vi "SwerveJoystickRotationScaling.vi"(2 "Rotation Scaling":dbl(slide)=2.0 min=1.0 max=4.0 scale=1.0..4.0, 3 "Rotation Deadband":dbl(slide)=0.05 min=0.0 max=0.4 scale=0.0..0.4, 4 "Auto Control":bool, 5 "Raw Rotation Joystick":dbl) -> (0 "Scaled Rotation Joystick":dbl, 1 "In Deadband":bool)   [LabVIEW 2019]
doc: "Applies a deadband and nonlinear scaling to the rotation axis of a swerve drive. Includes a hook to override the non-linear deadband and scaling when the rotation is under autonomous control."
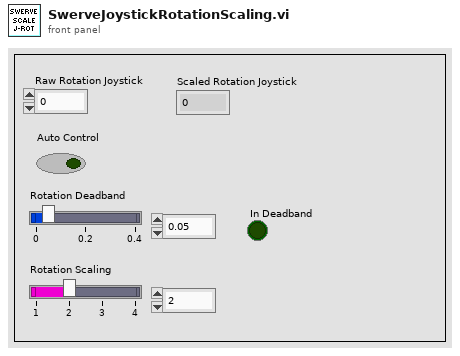
[diagram p1: front panel]
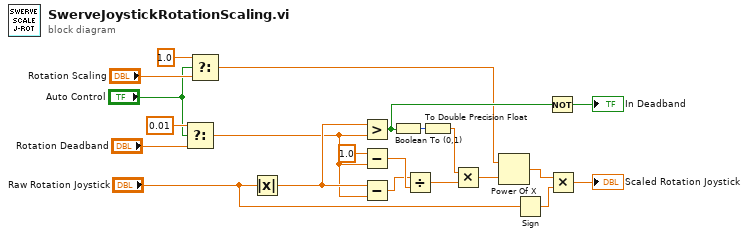
[diagram p0: block diagram]
diagram:
  n1 = Select(t=0.01, s="Auto Control", f="Rotation Deadband") -> (s? t:f=w5:dbl)
  n2 = Select(t=1.0, s="Auto Control", f="Rotation Scaling") -> (s? t:f=w2:dbl)
  n3 = Absolute Value(x="Raw Rotation Joystick") -> (abs(x)=w17:dbl)
  n4 = Greater?(x=w17, y=w5) -> (0:w18:bool)
  n5 = Subtract(x=1.0, y=w5) -> (x-y=w13:dbl)
  n6 = Subtract(x=w17, y=w5) -> (x-y=w11:dbl)
  n7 = Boolean To (0,1)(Boolean=w18) -> (0, 1=w9:i16)
  n8 = Divide(x=w11, y=w13) -> (x/y=w14:dbl)
  n9 = To Double Precision Float(number=w9) -> (double precision float=w10:dbl)
  n10 = Multiply(x=w10, y=w14) -> (x*y=w20:dbl)
  n11 = Power Of X(1:w20, 2:w2) -> (0:w21:dbl)
  n12 = Sign(1:"Raw Rotation Joystick") -> (0:w16:dbl)
  n13 = Not(x=w18) -> (.not. x?=→"In Deadband":bool)
  n14 = Multiply(x=w21, y=w16) -> (x*y=→"Scaled Rotation Joystick":dbl)
